vi "Query Target Relay.vi"(8 "error in":errorcluster, 10 "Relay Name":string, 11 "SwitchMatrix in":refnum<class "SwitchMatrix.lvclass">) -> (0 "error out":errorcluster, 2 "State":bool, 3 "SwitchMatrix out":refnum<class "SwitchMatrix.lvclass">)   [LabVIEW 2019, in "SwitchMatrix.lvlib" / "SwitchMatrix.lvclass"]
uses:
  Library/SwitchMatrix.lvclass
  Library/SwitchMatrix.lvclass/SwitchMatrix.ctl
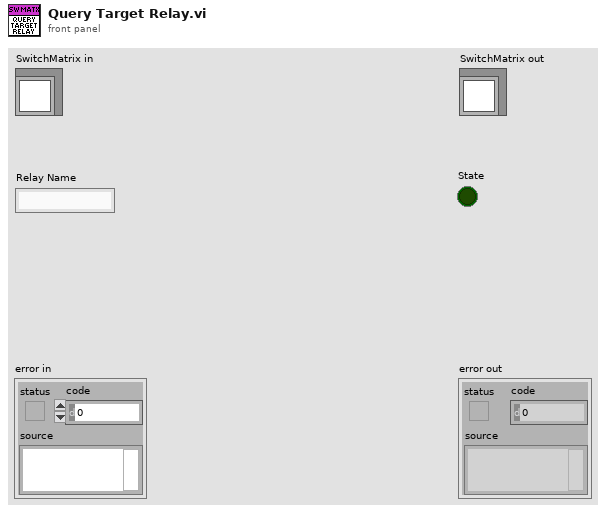
[diagram p1: front panel]
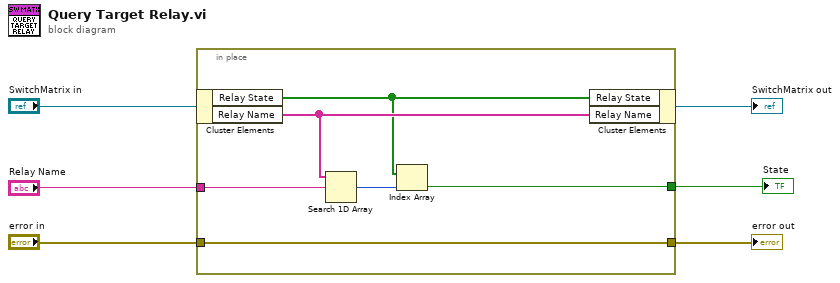
[diagram p0: block diagram]
diagram:
  n1 = in-place {
    in-place-border: "Relay Name" -> [w11]
    in-place-border: [w8] -> w3
    in-place-border: "error in" -> [w7]
    in-place-border: [w7] -> w1
    n2 = in-place-cluster #1("SwitchMatrix in") -> ("Relay State"=w9:bool[], "Relay Name"=w12:string[])
    n3 = Search 1D Array(1D array=w12, element=w11) -> (index of element=w10:i32)  [unwired: 1 in]
    n4 = Index Array(array=w9, index=w10) -> (element=w8:bool)
    n5 = in-place-cluster #1("Relay State"=w9, "Relay Name"=w12) -> (→"SwitchMatrix out":refnum<class "SwitchMatrix.lvclass">)
  }
  "error out" <- w1
  "State" <- w3
